vi "Cmd Set Parameter Properties (CR).vi"(4 "error in (no error)":errorcluster, 5 "parameter properties":T1, 6 "parameter index":variant, 7 "command-recordset reference":T4) -> (0 "error out":errorcluster, 3 "command-recordset reference out":T4)   [LabVIEW 2020, in "NI_Database_API.lvlib"]
doc: "Sets properties on the object as determined by the inputs. Wire data to the reference and properties inputs to determine the polymorphic instance to use or manually select the instance."
uses:
  <vilib>/addons/database/NI_Database_API.lvlib
  <vilib>/addons/database/Command-Recordset.llb/Cmd-Rec Object Reference.ctl
  <vilib>/addons/database/Command.llb/Cmd Parameter Properties.ctl
  <vilib>/addons/database/Auxilliary.llb/DB Tools DataTypes.ctl
  <vilib>/addons/database/Auxilliary.llb/DB Tools Parameter Dir.ctl
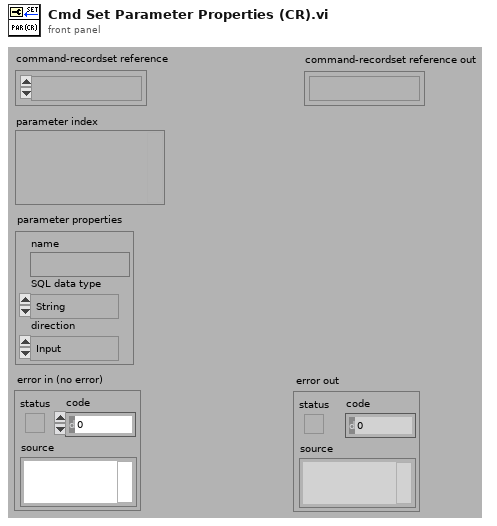
[diagram p1: front panel]
types:
  T1 = typedef "NI_Database_API.lvlib/Cmd Parameter Properties.ctl" = cluster{"name":string, "SQL data type":T2, "direction":T3}
  T2 = typedef "NI_Database_API.lvlib/DB Tools DataTypes.ctl" = enum16{"String", "Long (I32)", "Single (SGL)", "Double (DBL)", "Date/Time", "Binary"}
  T3 = typedef "NI_Database_API.lvlib/DB Tools Parameter Dir.ctl" = enum32{"Input", "Output", "Input/Output", "Return Value"}
  T4 = typedef "NI_Database_API.lvlib/Cmd-Rec Object Reference.ctl" = refnum<k1>
  T5 = typedef "NI_Database_API.lvlib/Cmd-Rec Data Members.ctl" = cluster{"recordset reference":T6, "command reference":T7}
  T6 = typedef "NI_Database_API.lvlib/Rec ObjectReference.ctl" = refnum<k1>
  T7 = typedef "NI_Database_API.lvlib/Cmd ObjectReference.ctl" = refnum<k1>
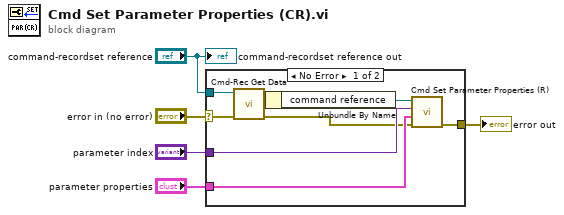
[diagram p0: block diagram]
diagram:
  n1 = case shown="No Error" "error in (no error)" {
    selector: "error in (no error)" -> [w6 w14]
    tunnel: [w13 w14] -> w5
    tunnel: "parameter index" -> [w12 _]
    tunnel: "parameter properties" -> [w11 _]
    tunnel: "command-recordset reference" -> [w7 _]
    frame No Error {
      n2 = call <vilib>:"Cmd-Rec Get Data.vi"("error in (no error)"=w6, "command-recordset reference"=w7) -> ("error out"=w8:errorcluster, "data"=w9:T5)  [unwired: 2 in, 2 out]
      n3 = Unbundle By Name(w9) -> ("command reference"=w10:T7)
      n4 = call <vilib>:"Cmd Set Parameter Properties (R).vi"("error in (no error)"=w8, "parameter properties"=w11, "parameter index"=w12, "command reference"=w10) -> ("error out"=w13:errorcluster)  [unwired: 2 in, 1 out]
    }
    frame Error {
    }
  }
  "error out" <- w5
  "command-recordset reference out" <- "command-recordset reference"
